vi "User Console - Init.vi"(8 "error in (no error)":errorcluster, 11 "User Console View":T1) -> (0 "error out":errorcluster, 3 "User Console View":T1)   [LabVIEW 2013]
doc: "Initializes the user console interface."
uses:
  Controls/User Console View.ctl
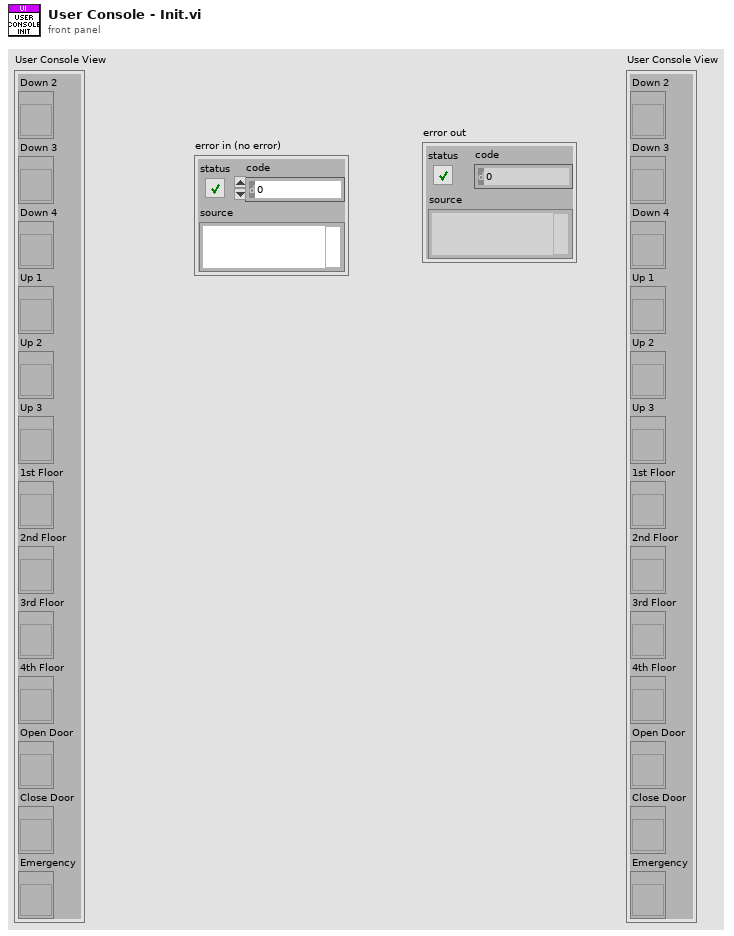
[diagram p1: front panel]
types:
  T1 = typedef "User Console View.ctl" = cluster{"Down 2":refnum<vi>, "Down 3":refnum<vi>, "Down 4":refnum<vi>, "Up 1":refnum<vi>, "Up 2":refnum<vi>, "Up 3":refnum<vi>, "1st Floor":refnum<vi>, "2nd Floor":refnum<vi>, "3rd Floor":refnum<vi>, "4th Floor":refnum<vi>, "Open Door":refnum<vi>, "Close Door":refnum<vi>, "Emergency":refnum<vi>}
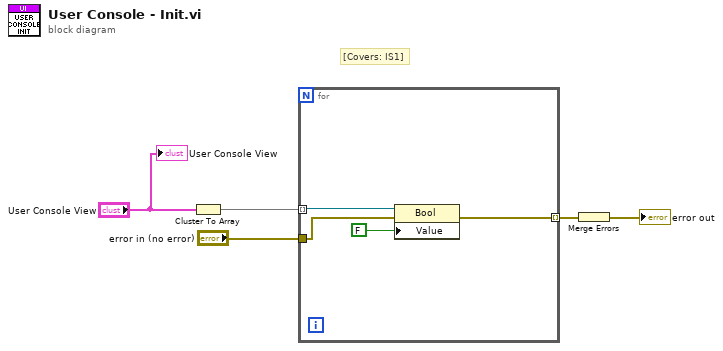
[diagram p0: block diagram]
diagram:
  # "[Covers: IS1]"
  n1 = Cluster To Array(cluster="User Console View") -> (array=w5:refnum<vi>[])
  n2 = for {
    tunnel: w5 -> [w9] mode=indexing
    tunnel: "error in (no error)" -> [w7]
    tunnel: [w6] -> w3 mode=indexing
    n3 = property class="Bool"(reference=w9, error in=w7, "Value"=FALSE) -> (error out=w6:errorcluster)  [unwired: 1 out]
  }
  n4 = Merge Errors(w3) -> (→"error out":errorcluster)
  "User Console View" <- "User Console View"
